vi "SN_parser.vi"(8 "error in (no error)":errorcluster, 10 "rules list":string[][](array[string]), 11 "SN in":string) -> (0 "error out":errorcluster, 2 "SN data":T1)   [LabVIEW 2024]
doc: "Empty State Machine"
uses:
  controls/SN_parser_data_cluster.ctl
  libraries/EV QSM support/support/queue state & data (Single).vi
  <vilib>/Utility/error.llb/Error Cluster From Error Code.vi
  <vilib>/ErrorRing/Error Ring.xnode
  libraries/EV QSM support/Ev Queued SM API.lvlib
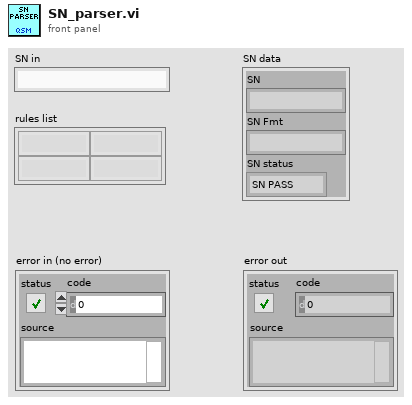
[diagram p1: front panel]
types:
  T1 = cluster{"SN":string, "SN Fmt":string, "SN status":enum16{"SN PASS", "SN FAIL"}}
  T2 = typedef "SN_parser_data_cluster.ctl" = cluster{"match?":bool, "Serial Number":string, "SN Fmt":string, "min_length":string, "max_length":string, "SN status":enum16{"SN PASS", "SN FAIL"}}
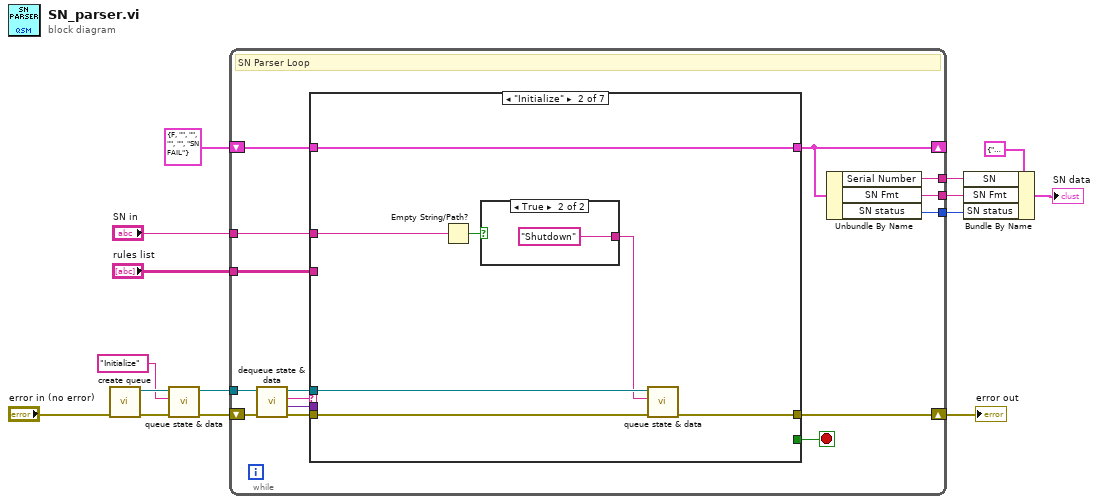
[diagram p0: block diagram]
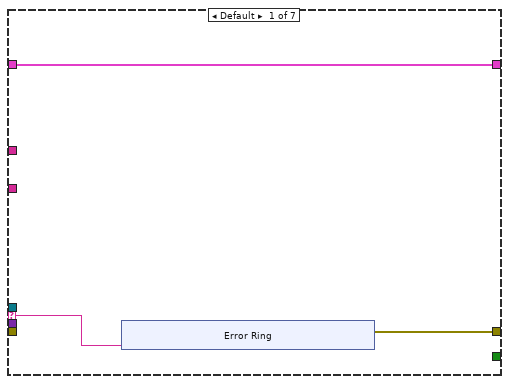
[diagram p2: hidden frame]
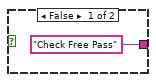
[diagram p3: hidden frame]
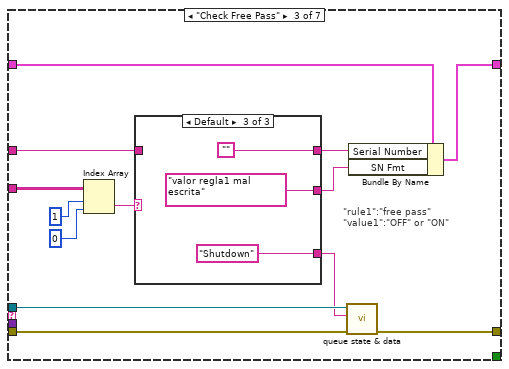
[diagram p4: hidden frame]
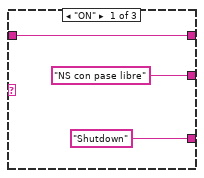
[diagram p5: hidden frame]
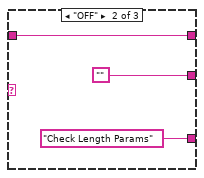
[diagram p6: hidden frame]
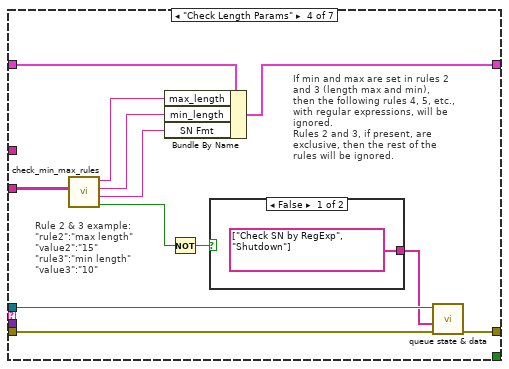
[diagram p7: hidden frame]
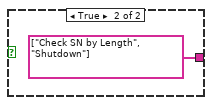
[diagram p8: hidden frame]
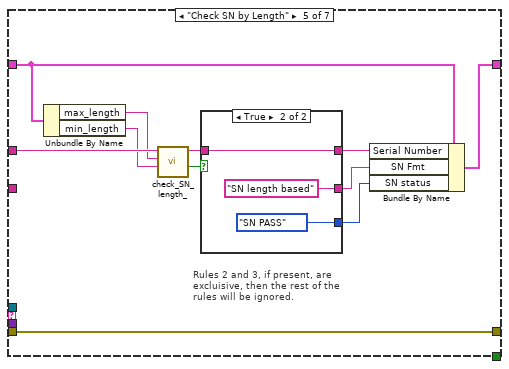
[diagram p9: hidden frame]
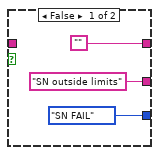
[diagram p10: hidden frame]
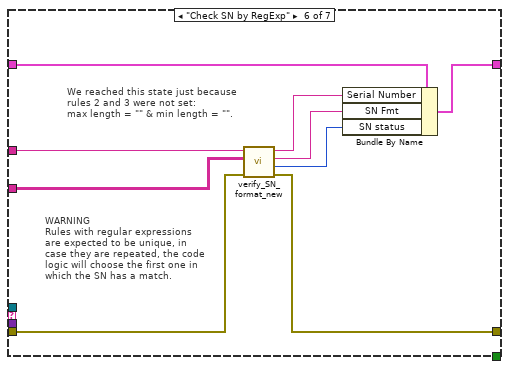
[diagram p11: hidden frame]
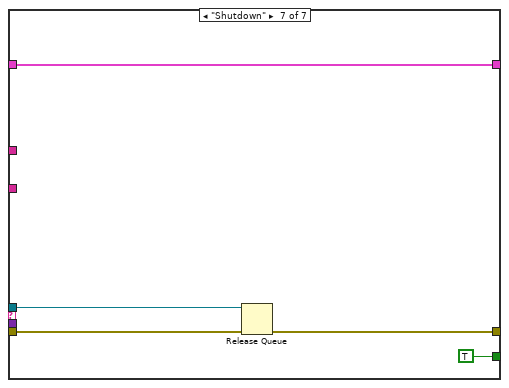
[diagram p12: hidden frame]
diagram:
  n1 = call "create queue.vi"("error in (no error)"="error in (no error)") -> ("error out"=w4:errorcluster, "queue out"=w15:refnum<queue>)  [unwired: 9 in]
  n2 = call-poly "queue state & data.vi"("error in (no error)"=w4, "State"="Initialize", "queue in"=w15) -> ("error out"=w3:errorcluster, "queue out"=w1:refnum<queue>)  [unwired: 7 in]
  n3 = while {
    shift-right: [w25] -> _
    shift-left: T2 {"match?"=FALSE, "Serial Number"="", "SN Fmt"="", "min_length"="", "max_length"="", "SN status"=enum."SN FAIL"} ("Data") -> [w29]
    shift-right: [w28] -> w13
    shift-left: w3 -> [w21]
    tunnel: "SN in" -> [w27]
    tunnel: "rules list" -> [w26]
    tunnel: [w24] -> w9
    tunnel: [w23] -> w8
    tunnel: [w22] -> w7
    tunnel: w1 -> [w19]
    stop <- w30 stop-if-true
    # "SN Parser Loop"
    n4 = call "dequeue state & data.vi"("error in (no error)"=w21, "queue in"=w19) -> ("error out"=w20:errorcluster, "State Data"=w16:variant, "State"=w17:string, "queue out"=w18:refnum<queue>)  [unwired: 6 in]
    n5 = case shown="\"Initialize\"" w17 {
      selector: w17 -> [w31 _ _ _ _ _ _]
      tunnel: [_ _ _ _ _ _ TRUE] -> w30
      tunnel: w29 -> [w33 w46 w54 w83 w90 w111 w116]
      tunnel: [w33 w46 w60 w82 w96 w110 w116] -> w25
      tunnel: w20 -> [_ w43 w52 w77 w86 w107 w113]
      tunnel: [w32 w42 w51 w76 w86 w106 w112] -> w28
      tunnel: w27 -> [_ w45 w55 _ w91 w108 _]
      tunnel: w26 -> [_ _ w57 w78 _ w109 _]
      tunnel: w18 -> [_ w47 w62 w73 _ _ w114]
      tunnel: w16 -> [_ _ _ _ _ _ _]
      frame Default {
        n6 = xnode "Error Ring"("parameter 0"=w31) -> ("error out"=w32:errorcluster)
      }
      frame "Initialize" {
        n7 = Empty String/Path?(string/path=w45) -> (empty?=w44:bool)
        n8 = case shown="True" w44 {
          tunnel: ["Check Free Pass" "Shutdown"] -> w41
          frame False {
          }
          frame True {
          }
        }
        n9 = call-poly "queue state & data.vi"("error in (no error)"=w43, "State"=w41, "queue in"=w47) -> ("error out"=w42:errorcluster)  [unwired: 7 in, 1 out]
      }
      frame "Check Free Pass" {
        # "\"rule1\":\"free pass\"\n\"value1\":\"OFF\" or \"ON\""
        n10 = Index Array(array=w57, index (row)=1 ("index"), index (col)=0 ("disabled index (col)")) -> (element=w56:string)
        n11 = case shown="Default" w56 {
          tunnel: [w65 w68 ""] -> w59
          tunnel: ["NS con pase libre" "" "valor regla1 mal escrita"] -> w58
          tunnel: w55 -> [w65 w68 _]
          tunnel: ["Shutdown" "Check Length Params" "Shutdown"] -> w50
          frame "ON" {
          }
          frame "OFF" {
          }
          frame Default {
          }
        }
        n12 = call-poly "queue state & data.vi"("error in (no error)"=w52, "State"=w50, "queue in"=w62) -> ("error out"=w51:errorcluster)  [unwired: 7 in, 1 out]
        n13 = Bundle By Name(cluster=w54, "Serial Number"=w59, "SN Fmt"=w58) -> (w60:T2)
      }
      frame "Check Length Params" {
        # "Rule 2 & 3 example:\n\"rule2\":\"max length\"\n\"value2\":\"15\"\n\"rule3\":\"min length\"\n\"value3\":\"10\""
        # "If min and max are set in rules 2 \nand 3 (length max and min), \nthen the following rules 4, 5, etc., \nwith regular expressions, will be\nignored.\nRules 2 and 3, if present, are\nexclusive, then the rest of the \nrules will be ignored."
        n14 = call "check_min_max_rules.vi"("rules list"=w78) -> ("empty/wrong?"=w74:bool, "message"=w81:string, "min_length"=w79:string, "max_length"=w80:string)  [unwired: 7 in]
        n15 = Bundle By Name(cluster=w83, "max_length"=w80, "min_length"=w79, "SN Fmt"=w81) -> (w82:T2)
        n16 = Not(x=w74) -> (.not. x?=w75:bool)
        n17 = case shown="False" w75 {
          tunnel: [string[] ["Check SN by RegExp", "Shutdown"] string[] ["Check SN by Length", "Shutdown"]] -> w72
          frame False {
          }
          frame True {
          }
        }
        n18 = call-poly "queue state & data.vi"("error in (no error)"=w77, "State Data"=w72, "queue in"=w73) -> ("error out"=w76:errorcluster)  [unwired: 7 in, 1 out]
      }
      frame "Check SN by Length" {
        # "Rules 2 and 3, if present, are\nexcluisive, then the rest of the \nrules will be ignored."
        n19 = Unbundle By Name(w90) -> ("max_length"=w89:string, "min_length"=w88:string)
        n20 = call "check_SN_length_.vi"("min length"=w88, "max length"=w89, "SN in"=w91) -> ("in range?"=w92:bool, "SN out"=w93:string)  [unwired: 7 in]
        n21 = case shown="True" w92 {
          tunnel: w93 -> [_ w102]
          tunnel: ["" w102] -> w95
          tunnel: ["SN outside limits" "SN length based"] -> w94
          tunnel: [enum16{"SN PASS", "SN FAIL"}."SN FAIL" ("SN status") enum16{"SN PASS", "SN FAIL"}."SN PASS" ("SN status")] -> w87
          frame False {
          }
          frame True {
          }
        }
        n22 = Bundle By Name(cluster=w90, "Serial Number"=w95, "SN Fmt"=w94, "SN status"=w87) -> (w96:T2)
      }
      frame "Check SN by RegExp" {
        # "WARNING\nRules with regular expressions \nare expected to be unique, in \ncase they are repeated, the code\nlogic will choose the first one in\nwhich the SN has a match."
        # "We reached this state just because \nrules 2 and 3 were not set: \nmax length = \"\" & min length = \"\"."
        n23 = call "verify_SN_format_new.vi"("error in (no error)"=w107, "rules list"=w109, "SN in"=w108) -> ("error out"=w106:errorcluster, "SN status"=w103:enum16{"SN PASS", "SN FAIL"}, "message"=w104:string, "SN out"=w105:string)  [unwired: 5 in]
        n24 = Bundle By Name(cluster=w111, "Serial Number"=w105, "SN Fmt"=w104, "SN status"=w103) -> (w110:T2)
      }
      frame "Shutdown" {
        n25 = Release Queue(queue=w114, error in (no error)=w113) -> (error out=w112:errorcluster)  [unwired: 1 in, 2 out]
      }
    }
    n26 = Unbundle By Name(w25) -> ("Serial Number"=w24:string, "SN Fmt"=w23:string, "SN status"=w22:enum16{"SN PASS", "SN FAIL"})
  }
  "error out" <- w13
  n27 = Bundle By Name(cluster=T1 {"SN"="", "SN Fmt"="", "SN status"=enum."SN PASS"} ("input cluster"), "SN"=w9, "SN Fmt"=w8, "SN status"=w7) -> (→"SN data":T1)
